vi "Select Channel Names.vi"(8 "error in (no error)":errorcluster, 11 "2D Channel Params":string[][](array[string])) -> (0 "error out":errorcluster, 2 "Ch.Names":string[](array[string]), 3 "Ch.Description -1":string[](array[string]))   [LabVIEW 2017]
doc: "This SubVI select a 1D Array of channel names\nfrom 2D array of channle properties, and then\ndelete last element which is TimeStamp"
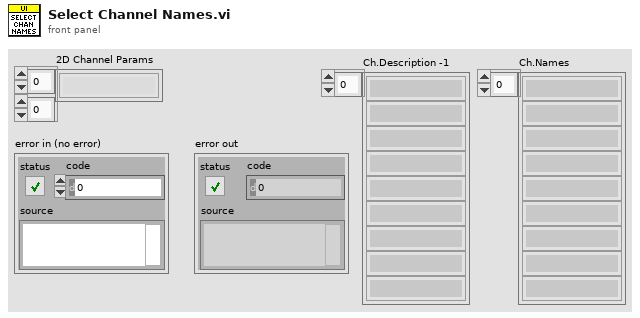
[diagram p1: front panel]
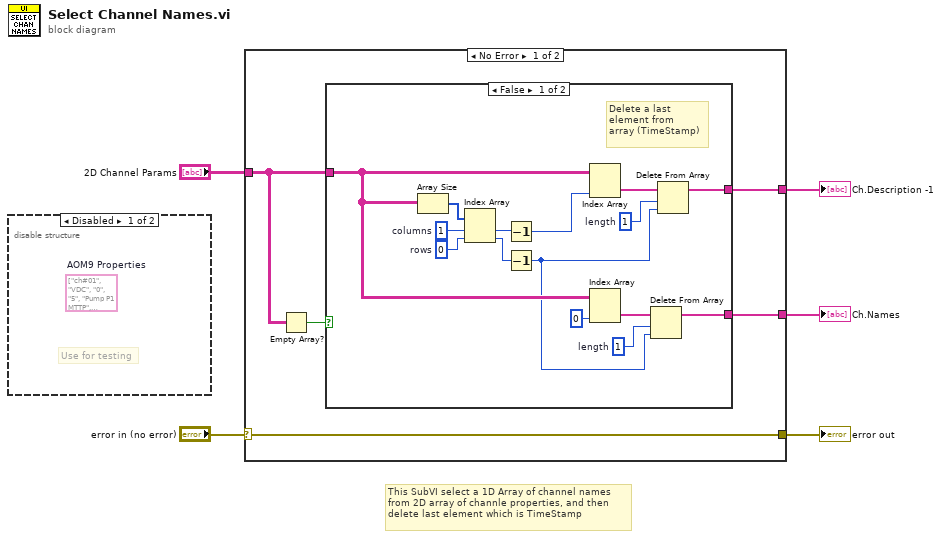
[diagram p0: block diagram]
diagram:
  # "This SubVI select a 1D Array of channel names\nfrom 2D array of channle properties, and then\ndelete last element which is TimeStamp"
  n1 = disable-structure shown="Disabled" {
    frame Disabled {
      (unwired) string[][] [["ch#01", "VDC", "0", "5", "Pump P1 MTTP"], ["ch#02", "VDC", "0", "5", "Pump P2 MTTP"], ["ch#03", "VDC", "0", "5", "Pump P3 MTTP"], ["ch#04", "VDC", "0", "5", "Pump P4 MTTP"], ["ch#05", "VDC", "0", "5", "Reserve AO1"], ["ch#06", "VDC", "0", "5", "Reserve AO2"], ["TimeStamp", "seconds", "", "", "Date & Time"]]  # AOM9 Properties
      # "Use for testing"
    }
    frame Enabled {
    }
  }
  n2 = case shown="No Error" "error in (no error)" {
    selector: "error in (no error)" -> [w10 w26]
    tunnel: [w10 w26] -> w4
    tunnel: "2D Channel Params" -> [w8 _]
    tunnel: [w9 _] -> w3
    tunnel: [w6 _] -> w2
    frame No Error {
      n3 = Empty Array?(array=w8) -> (empty?=w7:bool)
      n4 = case shown="False" w7 {
        tunnel: [w18 _] -> w9
        tunnel: w8 -> [w16 _]
        tunnel: [w11 _] -> w6
        frame False {
          w14 = 1  # length
          w19 = 1  # length
          w20 = 0  # rows
          w24 = 1  # columns
          # "Delete a last\nelement from\narray (TimeStamp)"
          n5 = Array Size(array=w16) -> (size(s)=w25:i32[])
          n6 = Index Array(array=w25, index #1=w24, index #2=w20) -> (element #1=w23:i32, element #2=w17:i32)
          n7 = Decrement(x=w23) -> (x-1=w22:i32)
          n8 = Decrement(x=w17) -> (x-1=w12:i32)
          n9 = Index Array(array=w16, index (col)=w22) -> (element=w21:string[])  [unwired: 1 in]
          n10 = Index Array(array=w16, index (col)=0 ("disabled index (col)")) -> (element=w13:string[])  [unwired: 1 in]
          n11 = Delete From Array(array=w13, length=w14, index=w12) -> (array with subset deleted=w11:string[])  [unwired: 1 out]
          n12 = Delete From Array(array=w21, length=w19, index=w12) -> (array with subset deleted=w18:string[])  [unwired: 1 out]
        }
        frame True {
          # "If this is empty array Do nothing"
        }
      }
    }
    frame Error {
    }
  }
  "error out" <- w4
  "Ch.Description -1" <- w3
  "Ch.Names" <- w2
